vi "ClimbNetwork.vi"   [LabVIEW 2023]
uses:
  ClimbNetworkingGlobal.vi
  <vilib>/Rock Robotics/Network Tables/NT Write Boolean.vi
  <vilib>/Rock Robotics/Network Tables/NT Write Number.vi
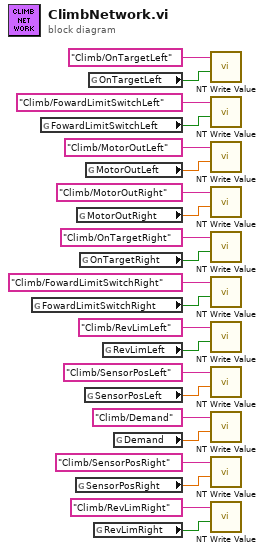
[diagram p0: block diagram]
diagram:
  n1 = global read "ClimbNetworkingGlobal.vi" "FowardLimitSwitchRight"() -> (w11:bool)
  n2 = global read "ClimbNetworkingGlobal.vi" "FowardLimitSwitchLeft"() -> (w19:bool)
  n3 = global read "ClimbNetworkingGlobal.vi" "SensorPosRight"() -> (w3:dbl)
  n4 = global read "ClimbNetworkingGlobal.vi" "MotorOutRight"() -> (w15:dbl)
  n5 = global read "ClimbNetworkingGlobal.vi" "OnTargetRight"() -> (w13:bool)
  n6 = global read "ClimbNetworkingGlobal.vi" "SensorPosLeft"() -> (w7:dbl)
  n7 = global read "ClimbNetworkingGlobal.vi" "MotorOutLeft"() -> (w17:dbl)
  n8 = global read "ClimbNetworkingGlobal.vi" "OnTargetLeft"() -> (w21:bool)
  n9 = global read "ClimbNetworkingGlobal.vi" "RevLimRight"() -> (w1:bool)
  n10 = global read "ClimbNetworkingGlobal.vi" "RevLimLeft"() -> (w9:bool)
  n11 = global read "ClimbNetworkingGlobal.vi" "Demand"() -> (w5:dbl)
  n12 = call-poly <vilib>:"NT Write Value.vi"("value"=w21, "name"="Climb/OnTargetLeft") -> ()  [unwired: 9 in, 1 out]
  n13 = call-poly <vilib>:"NT Write Value.vi"("value"=w19, "name"="Climb/FowardLimitSwitchLeft") -> ()  [unwired: 9 in, 1 out]
  n14 = call-poly <vilib>:"NT Write Value.vi"("value"=w17, "name"="Climb/MotorOutLeft") -> ()  [unwired: 9 in, 1 out]
  n15 = call-poly <vilib>:"NT Write Value.vi"("value"=w15, "name"="Climb/MotorOutRight") -> ()  [unwired: 9 in, 1 out]
  n16 = call-poly <vilib>:"NT Write Value.vi"("value"=w13, "name"="Climb/OnTargetRight") -> ()  [unwired: 9 in, 1 out]
  n17 = call-poly <vilib>:"NT Write Value.vi"("value"=w11, "name"="Climb/FowardLimitSwitchRight") -> ()  [unwired: 9 in, 1 out]
  n18 = call-poly <vilib>:"NT Write Value.vi"("value"=w9, "name"="Climb/RevLimLeft") -> ()  [unwired: 9 in, 1 out]
  n19 = call-poly <vilib>:"NT Write Value.vi"("value"=w7, "name"="Climb/SensorPosLeft") -> ()  [unwired: 9 in, 1 out]
  n20 = call-poly <vilib>:"NT Write Value.vi"("value"=w5, "name"="Climb/Demand") -> ()  [unwired: 9 in, 1 out]
  n21 = call-poly <vilib>:"NT Write Value.vi"("value"=w3, "name"="Climb/SensorPosRight") -> ()  [unwired: 9 in, 1 out]
  n22 = call-poly <vilib>:"NT Write Value.vi"("value"=w1, "name"="Climb/RevLimRight") -> ()  [unwired: 9 in, 1 out]
